vi "Job Message To Data.vi"(8 "Error In":errorcluster, 11 "Job Message":string) -> (0 "Error Out":errorcluster, 2 "LabVIEW Version":T1, 3 "Job Source File Name":string)   [LabVIEW 2013, in "LVH-Revert.lvlib"]
uses:
  LVH-Revert.lvlib
  <vilib>/LabVIEW Hacker/LVH-Toolbox/Common/Private/Type Defs/LabVIEW Version.ctl
  <vilib>/LabVIEW Hacker/LVH-Toolbox/Common/LVH-Common.lvlib
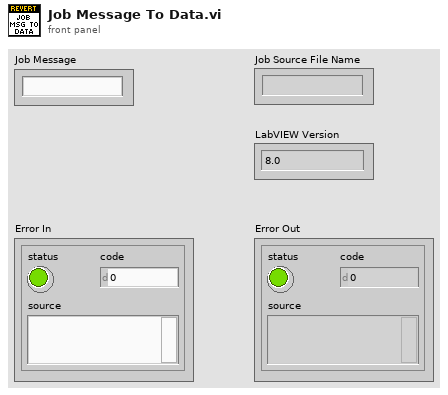
[diagram p1: front panel]
types:
  T1 = typedef "LVH-Toolbox.lvlib/LVH-Common.lvlib/LabVIEW Version.ctl" = enum16{"8.0", "8.2", "8.6", "9.0", "10.0", "11.0", "12.0", "13.0"}
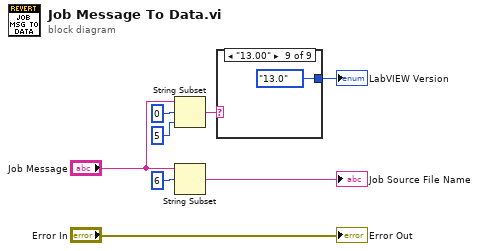
[diagram p0: block diagram]
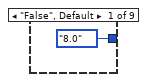
[diagram p2: hidden frame]
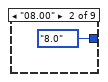
[diagram p3: hidden frame]
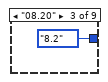
[diagram p4: hidden frame]
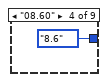
[diagram p5: hidden frame]
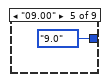
[diagram p6: hidden frame]
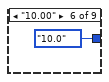
[diagram p7: hidden frame]
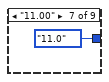
[diagram p8: hidden frame]
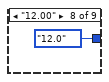
[diagram p9: hidden frame]
diagram:
  n1 = String Subset(string="Job Message", offset (0)=0, length (rest)=5 ("length (rest)")) -> (substring=w3:string)
  n2 = String Subset(string="Job Message", offset (0)=6 ("length (rest)")) -> (substring=→"Job Source File Name":string)  [unwired: 1 in]
  n3 = case shown="\"13.00\"" w3 {
    tunnel: [LabVIEW_Version."8.0" ("LabVIEW Version") LabVIEW_Version."8.0" ("LabVIEW Version") LabVIEW_Version."8.2" ("LabVIEW Version") LabVIEW_Version."8.6" ("LabVIEW Version") LabVIEW_Version."9.0" ("LabVIEW Version") LabVIEW_Version."10.0" ("LabVIEW Version") LabVIEW_Version."11.0" ("LabVIEW Version") LabVIEW_Version."12.0" ("LabVIEW Version") LabVIEW_Version."13.0" ("LabVIEW Version")] -> w2
    frame "False", Default {
    }
    frame "08.00" {
    }
    frame "08.20" {
    }
    frame "08.60" {
    }
    frame "09.00" {
    }
    frame "10.00" {
    }
    frame "11.00" {
    }
    frame "12.00" {
    }
    frame "13.00" {
    }
  }
  "LabVIEW Version" <- w2
  "Error Out" <- "Error In"
